vi "Get Message.vi"(8 "error in (no error)":errorcluster, 11 "SPARC4_GUI in":refnum<class "SPARC4_GUI.lvclass">) -> (0 "error out":errorcluster, 3 "SPARC4_GUI out":refnum<class "SPARC4_GUI.lvclass">)   [LabVIEW 2018, in "SPARC4_GUI.lvclass"]
uses:
  SPARC4_GUI.lvclass
  SPARC4_GUI.lvclass/SPARC4_GUI.ctl
  Stream/Stream.lvclass
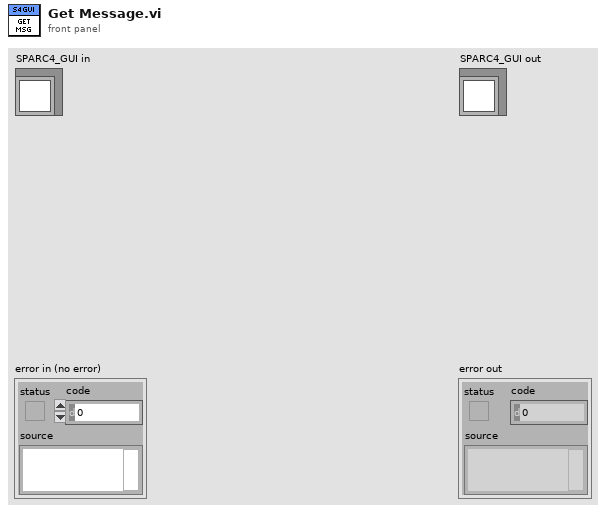
[diagram p1: front panel]
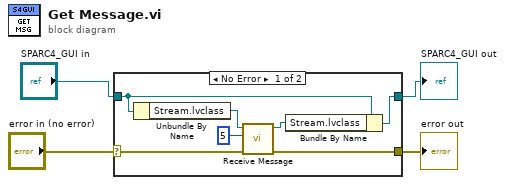
[diagram p0: block diagram]
diagram:
  n1 = case shown="No Error" "error in (no error)" {
    selector: "error in (no error)" -> [w11 w13]
    tunnel: [w10 w13] -> w3
    tunnel: [w6 w12] -> w1
    tunnel: "SPARC4_GUI in" -> [w8 w12]
    frame No Error {
      n2 = Unbundle By Name(w8) -> ("Stream.lvclass"=w9:refnum<class "Stream.lvclass">)
      n3 = call "Receive Message.vi"("error in (no error)"=w11, "timeout ms"=5, "Stream in"=w9) -> ("error out"=w10:errorcluster, "Stream out"=w7:refnum<class "Stream.lvclass">)  [unwired: 7 in]
      n4 = Bundle By Name(cluster=w8, "Stream.lvclass"=w7) -> (w6:refnum<class "SPARC4_GUI.lvclass">)
    }
    frame Error {
    }
  }
  "error out" <- w3
  "SPARC4_GUI out" <- w1
